vi "Backup.vi"(8 "error in":errorcluster, 11 "Auto Notifiers In":T1) -> (0 "error out":errorcluster, 3 "Auto Notifiers Out":T1)   [LabVIEW 2014]
uses:
  Auto Notifiers.ctl
  Main/Arms/Arm clapper state.ctl
  Main/Arms/Arm State.ctl
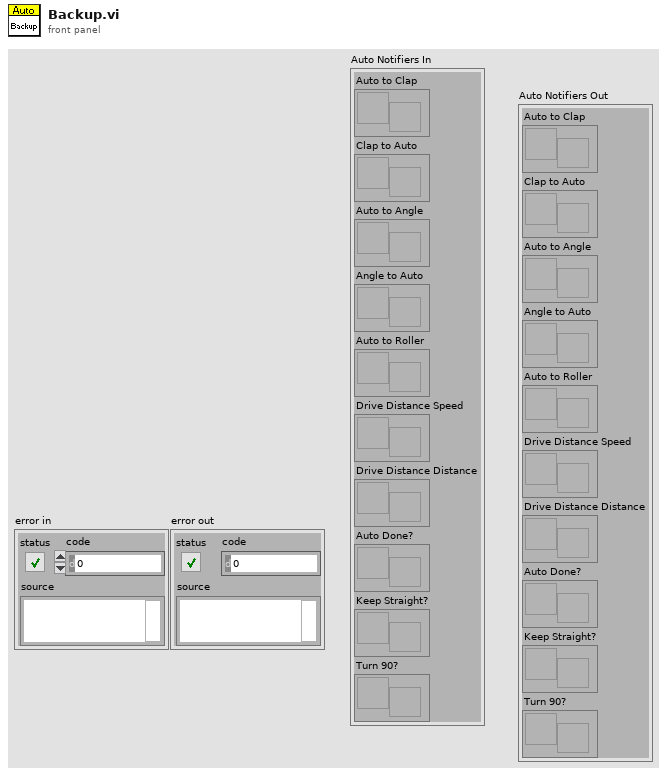
[diagram p1: front panel]
types:
  T1 = typedef "Auto Notifiers.ctl" = cluster{"Auto to Clap":refnum<notifier>, "Clap to Auto":refnum<notifier>, "Auto to Angle":refnum<notifier>, "Angle to Auto":refnum<notifier>, "Auto to Roller":refnum<notifier>, "Drive Distance Speed":refnum<notifier>, "Drive Distance Distance":refnum<notifier>, "Auto Done?":refnum<notifier>, "Keep Straight?":refnum<notifier>, "Turn 90?":refnum<notifier>}
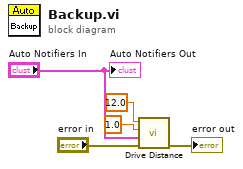
[diagram p0: block diagram]
diagram:
  n1 = call "Drive Distance.vi"("error in"="error in", "Auto Notifiers In"="Auto Notifiers In", "Speed"=1.0, "Distance (inches)"=12.0) -> ("error out"=→"error out":errorcluster)  [unwired: 6 in, 1 out]
  "Auto Notifiers Out" <- "Auto Notifiers In"
